vi "gbl.vi"() -> ()   [LabVIEW 2018]
panel:
  in  "采样间隔ms":dbl
  in  "流道间隙mm":dbl
  in  "监测曲线平滑度":i32
  in  "报警信息":string[][](array[string])
  in  "单独采样":i32
  out "计算数据":dbl[][](array[numeric])
  out "特征点Y":dbl[](array[numeric])
  out "特征点X":dbl[](array[numeric])
  out "WaveData":dbl[][](array[numeric])
  out "WaveTime":dbl[](array[numeric])
  in  "数据保存路径":path
  in  "A数组":dbl[](array[numeric])
  in  "V数组":dbl[](array[numeric])
  in  "X数组":timestamp[](array[timestamp])
  in  "衰减下限":dbl
  in  "衰减上限":dbl
  in  "声速下限":dbl
  in  "声速上限":dbl
  in  "本次监测名称":string
  in  "采样深度":i32
  in  "当前通道号":u8
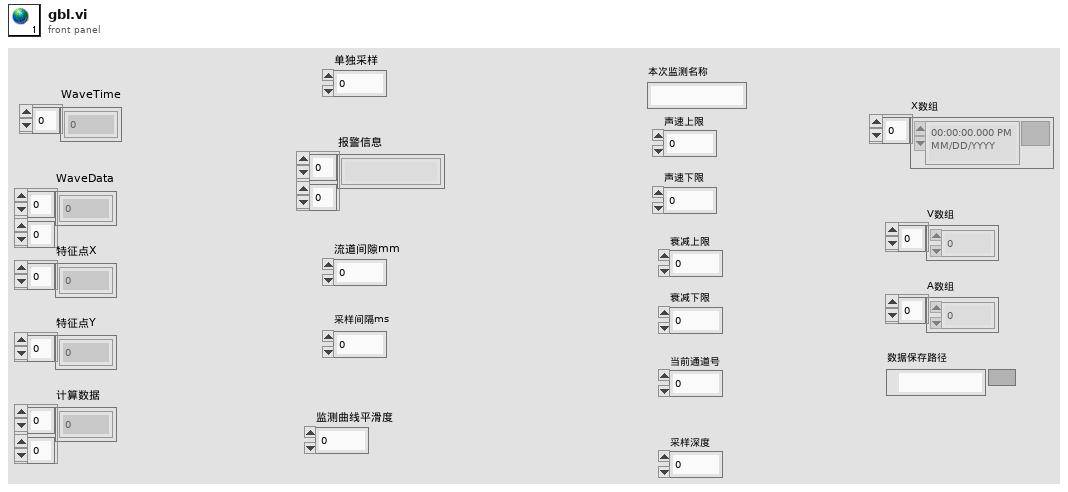
[diagram p1: front panel]
diagram:
